vi "Add VI Tree Item.vi"(8 "Error In":errorcluster, 10 "VI Tree Tag":string, 11 "TreeControl In":refnum<vi>) -> (0 "Error Out":errorcluster, 2 "VI Tree Tag":string, 3 "TreeControl Out":refnum<vi>)   [LabVIEW 2017, in "Bookmark Manager.lvlib"]
uses:
  Bookmark Manager.lvlib
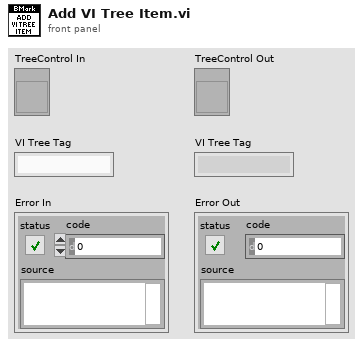
[diagram p1: front panel]
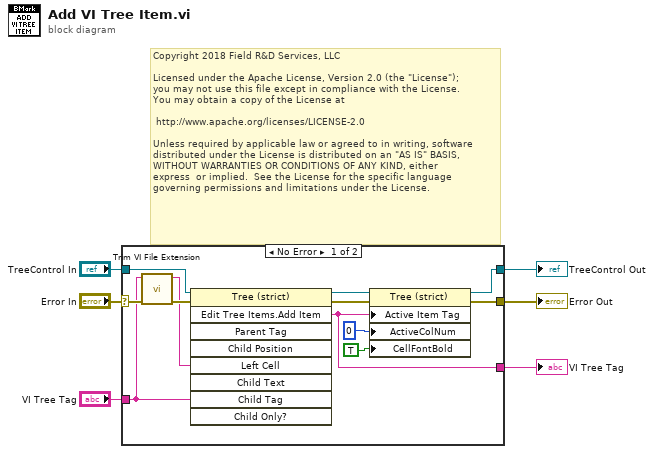
[diagram p0: block diagram]
diagram:
  # "Copyright 2018 Field R&D Services, LLC\n\nLicensed under the Apache License, Version 2.0 (the \"License\");\nyou may not use this file except in compliance with the License.\nYou may obtain a copy of the License at\n\n\thttp://www.apache.org/licenses/LICENSE-2.0\n\nUnless required by applicable law or agreed to in writing, software\ndistributed under the License is distributed on an \"AS IS\" BASIS,\nWITHOUT WARRANTIES OR CONDITIONS OF ANY KIND, either \nexpress  or implied.  See the License for the specific language \ngoverning permissions and limitations under the License."
  n1 = case shown="No Error" "Error In" {
    selector: "Error In" -> [w10 w20]
    tunnel: [w18 _] -> w6
    tunnel: [w14 w19] -> w5
    tunnel: "TreeControl In" -> [w12 w19]
    tunnel: [w11 w20] -> w3
    tunnel: "VI Tree Tag" -> [w8 _]
    frame No Error {
      n2 = call "Trim VI File Extension.vi"("Error In"=w10, "VI File Name"=w8) -> ("Error Out"=w9:errorcluster, "VI Name"=w7:string)  [unwired: 8 in]
      n3 = invoke class="Tree (strict)" method="Edit Tree Items.Add Item"(reference=w12, error in=w9, "Left Cell"=w7, "Child Tag"=w8) -> (reference out=w13:refnum<vi>, error out=w15:errorcluster, "Edit Tree Items:Add Item"=w18:string)  [unwired: 5 in, 6 out]
      n4 = property class="Tree (strict)"(reference=w13, error in=w15, "Active Item Tag"=w18, "ActiveColNum"=0 ("Active Cell:Active Column Number"), "CellFontBold"=TRUE ("Active Cell:Cell Font:Bold")) -> (reference out=w14:refnum<vi>, error out=w11:errorcluster)
    }
    frame Error {
    }
  }
  "Error Out" <- w3
  "VI Tree Tag" <- w6
  "TreeControl Out" <- w5
